vi "斯坦道XML解析.vi"(11 "参数簇":T1 {"启动参数" items=["总磷"=131, "总氮"=76, "总磷海水"=147, "总氮海水"=92]}) -> (2 "步骤时间":string[](array[string]), 3 "步骤名":string[](array[string]))   [LabVIEW 2016, in "总磷.lvlib"]
uses:
  <vilib>/Utility/sysdir.llb/System Directory Type.ctl
  <vilib>/xml/Load XML File.vi
  <vilib>/xml/Close Reference(Node).vi
  <resource>/objmgr/DOMUserDefRef.rc
  <vilib>/xml/NI_XML.lvlib
panel:
  out "添加的路径":path
  out "XML字符串":string="<?xml version=\"1.0\" encoding=\"ISO-8859-1\"?>\n<bookstore>\n<book ISBN=\"978-0545128285\">\n  <title lang=\"en\">The Tales of Beedle the Bard</title>\n  <author>J. K. Rowling</author>\n  <year>2008</year>\n  <price>12.99</price>\n</book>\n<book ISBN=\"978-0316160209\">\n  <title lang=\"en\">Eclipse</title>\n  <author>Stephenie Meyer</author>\n  <year>2007</year>\n  <price>19.99</price>\n</book>\n<book ISBN=\"978-0316067928\">\n  <title lang=\"en\">Breaking Dawn</title>\n  <author>Stephenie Meyer</author>\n  <year>2008</year>\n  <price>22.99</price>\n</book>\n<book ISBN=\"978-0316017923\">\n  <title lang=\"en\">Outliers: The Story of Success</title>\n  <author>Malcolm Gladwell</author>\n  <year>2008</year>\n  <price>27.99</price>\n</book>\n<book ISBN=\"978-0596007645\">\n  <title lang=\"en\">XML in a Nutshell</title>\n  <author>Elliotte Rusty Harold</author>\n  <author>W. Scott Means</author>\n  <year>2004</year>\n  <price>39.95</price>\n</book>\n</bookstore>"
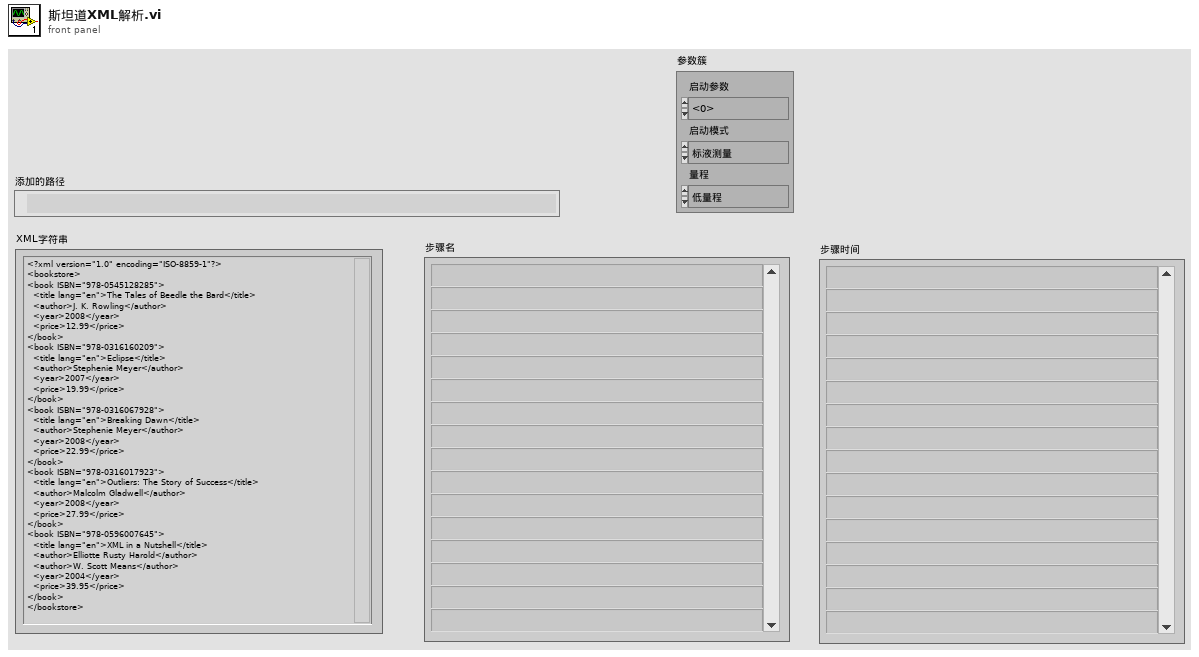
[diagram p1: front panel]
types:
  T1 = cluster{"启动模式":enum16{"标液测量", "水样测量", "零液测量", "盲样测量", "加标回收"}, "启动参数":u16, "量程":enum16{"低量程", "高量程"}}
  T2 = typedef "System Directory Type.ctl" = i32
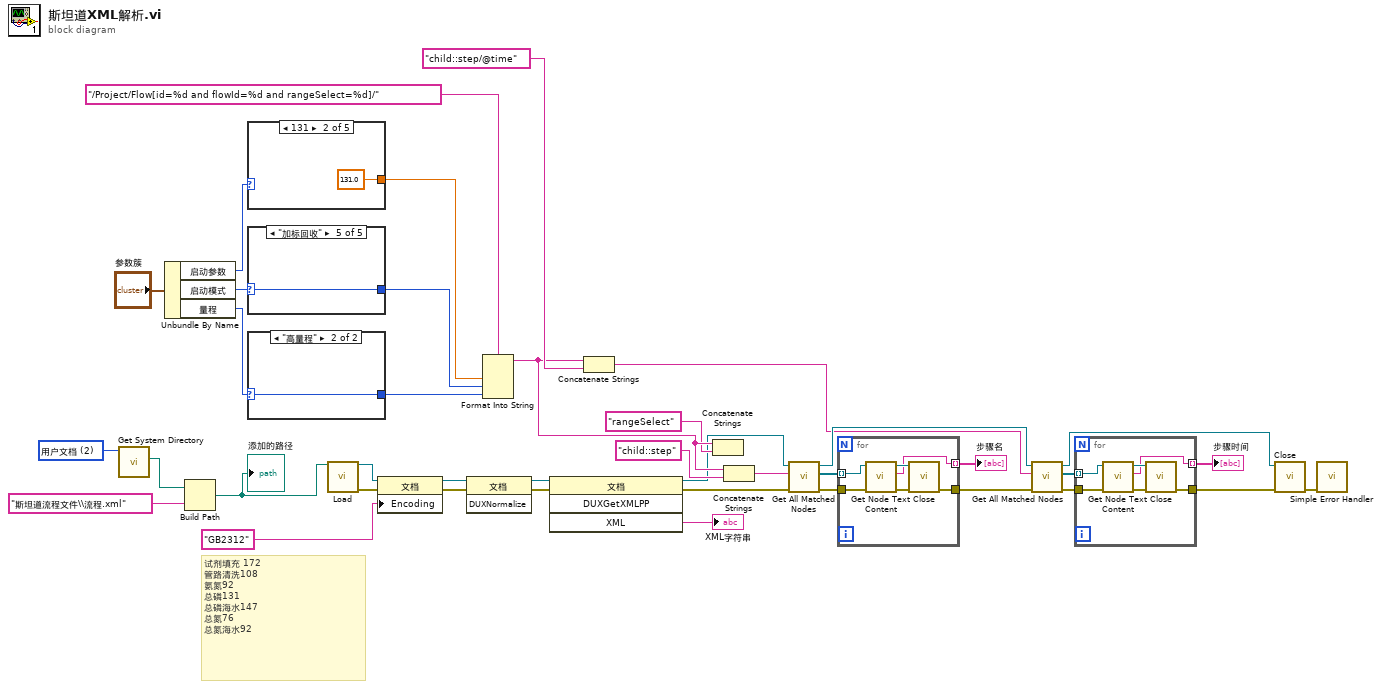
[diagram p0: block diagram]
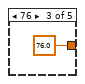
[diagram p8: hidden frame]
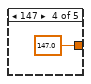
[diagram p9: hidden frame]
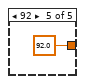
[diagram p10: hidden frame]
diagram:
  w31 = T2 2 items=["用户目录"=0, "用户桌面"=1, "用户文档"=2, "用户应用程序数据"=3, "用户设置"=4, "用户临时目录"=5, "公共文档"=6, "公共应用程序数据"=7, "公共设置"=8, "公共缓存"=13, "系统核心库"=9, "系统安装库"=10, "应用程序文件"=11, "启动盘根目录"=12] ("system directory type")
  # "试剂填充 172 \n管路清洗108\n氨氮92\n总磷131\n总磷海水147\n总氮76\n总氮海水92"
  n1 = call <vilib>:"Get System Directory.vi"("system directory type"=w31) -> ("system directory"=w30:path)  [unwired: 10 in]
  n2 = Unbundle By Name("参数簇") -> ("启动参数"=w3:u16, "启动模式"=w2:enum16{"标液测量", "水样测量", "零液测量", "盲样测量", "加标回收"}, "量程"=w1:enum16{"低量程", "高量程"})
  n3 = Build Path(base path=w30, name or relative path="斯坦道流程文件\\流程.xml" ("名称或相对路径")) -> (appended path=w28:path)
  "添加的路径" <- w28
  n4 = case shown="131" w3 {
    selector: w3 -> [w40 _ _ _ _]
    tunnel: [w40 131.0 ("输入 1") 76.0 ("输入 1") 147.0 ("输入 1") 92.0 ("输入 1")] -> w24
    frame Default {
    }
    frame 131 {
    }
    frame 76 {
    }
    frame 147 {
    }
    frame 92 {
    }
  }
  n5 = case shown="\"加标回收\"" w2 {
    selector: w2 -> [w45 w46 w47 w48 w49]
    tunnel: [w45 w46 w47 w48 w49] -> w23
    frame "标液测量", Default {
    }
    frame "水样测量" {
    }
    frame "零液测量" {
    }
    frame "盲样测量" {
    }
    frame "加标回收" {
    }
  }
  n6 = case shown="\"高量程\"" w1 {
    selector: w1 -> [w50 w51]
    tunnel: [w50 w51] -> w22
    frame "低量程", Default {
    }
    frame "高量程" {
    }
  }
  n7 = call-poly <vilib>:"Load.vi"("path to XML document"=w28) -> ("DOM document out"=w37:refnum<k20>, "error out"=w36:errorcluster)  [unwired: 12 in, 1 out]
  n8 = property on="属性节点" class="文档"(reference=w37, error in=w36, "Encoding"="GB2312" ("文档编码")) -> (reference out=w35:refnum<k20>, error out=w34:errorcluster)
  n9 = invoke on="Invoke Node" class="文档" method="DUXNormalize"(reference=w35, error in=w34) -> (reference out=w32:refnum<k20>, error out=w33:errorcluster)  [unwired: 1 in, 1 out]
  n10 = Format Into String(format string="/Project/Flow[id=%d and flowId=%d and rangeSelect=%d]/" ("XPath expression"), w24, w23, w22) -> (resulting string=w10:string)  [unwired: 2 in, 1 out]
  n11 = invoke on="Invoke Node" class="文档" method="DUXGetXMLPP"(reference=w32, error in=w33) -> (reference out=w6:refnum<k20>, error out=w7:errorcluster, "XML"=→"XML字符串":string)  [unwired: 2 in, 1 out]
  n12 = Concatenate Strings(w10, "child::step/@time" ("输入 4")) -> (w11:string)
  n13 = Concatenate Strings(w10, "rangeSelect" ("输入 4")) -> ()  [unwired: 1 out]
  n14 = Concatenate Strings(w10, "child::step" ("输入 4")) -> (w13:string)
  n15 = call <vilib>:"Get All Matched Nodes.vi"("error in (no error)"=w7, "XPath expression"=w13, "node in"=w6) -> ("error out"=w27:errorcluster, "node result array"=w26:refnum<k20>[], "node out"=w17:refnum<k20>)  [unwired: 6 in]
  n16 = for {
    tunnel: w27 -> [w57]
    tunnel: [w54] -> w21 mode=indexing
    tunnel: w26 -> [w53] mode=indexing
    tunnel: [w52] -> w16
    n17 = call <vilib>:"Get Node Text Content.vi"("error in (no error)"=w57, "node in"=w53) -> ("error out"=w55:errorcluster, "node text"=w54:string, "node out"=w56:refnum<k20>)  [unwired: 7 in]
    n18 = call-poly <vilib>:"Close.vi"("error in (no error)"=w55, "node"=w56) -> ("error out"=w52:errorcluster)  [unwired: 7 out]
  }
  "步骤名" <- w21
  n19 = call <vilib>:"Get All Matched Nodes.vi"("error in (no error)"=w16, "XPath expression"=w11, "node in"=w17) -> ("error out"=w19:errorcluster, "node result array"=w18:refnum<k20>[], "node out"=w5:refnum<k20>)  [unwired: 6 in]
  n20 = for {
    tunnel: w19 -> [w63]
    tunnel: [w60] -> w15 mode=indexing
    tunnel: w18 -> [w59] mode=indexing
    tunnel: [w58] -> w8
    n21 = call <vilib>:"Get Node Text Content.vi"("error in (no error)"=w63, "node in"=w59) -> ("error out"=w61:errorcluster, "node text"=w60:string, "node out"=w62:refnum<k20>)  [unwired: 7 in]
    n22 = call-poly <vilib>:"Close.vi"("error in (no error)"=w61, "node"=w62) -> ("error out"=w58:errorcluster)  [unwired: 7 out]
  }
  "步骤时间" <- w15
  n23 = call-poly <vilib>:"Close.vi"("error in (no error)"=w8, "node"=w5) -> ("error out"=w20:errorcluster)  [unwired: 7 out]
  n24 = call <vilib>:"Simple Error Handler.vi"("error in (no error)"=w20) -> ()  [unwired: 4 in, 5 out]
